vi "Count.vi"(0 "LV MDI in":refnum<class "LV MDI.lvclass">, 11 "error in (no error)":errorcluster) -> (4 "LV MDI out":refnum<class "LV MDI.lvclass">, 10 "Count":i32, 15 "error out":errorcluster)   [LabVIEW 2016, in "LV MDI.lvclass"]
doc: "Returns number of loaded vi."
uses:
  LV MDI.lvclass
  LV MDI.lvclass/LV MDI.ctl
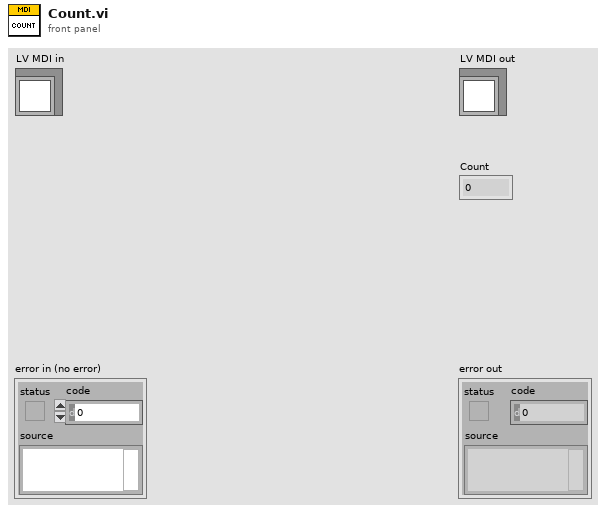
[diagram p1: front panel]
types:
  T1 = typedef "LV MDI.lvclass/Child Window Data.ctl" = cluster{"Child hWnd":u32, "UID":string, "vi reference":refnum<vi>, "Name":string}
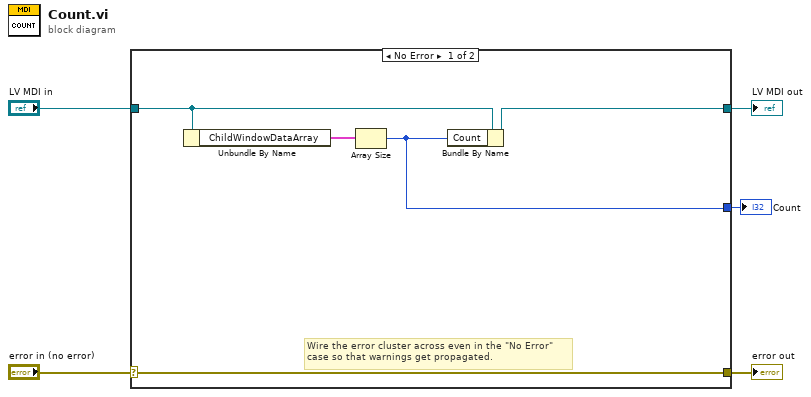
[diagram p0: block diagram]
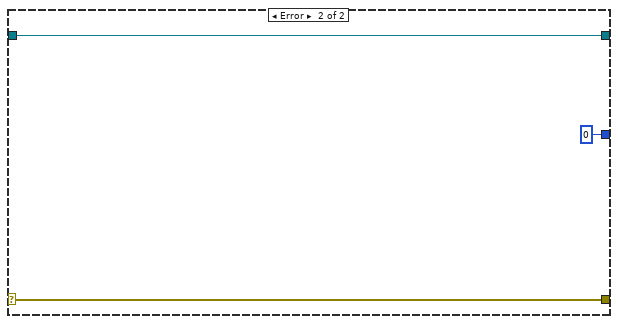
[diagram p2: hidden frame]
diagram:
  n1 = case shown="No Error" "error in (no error)" {
    selector: "error in (no error)" -> [w10 w13]
    tunnel: [w10 w13] -> w4
    tunnel: [w7 w12] -> w2
    tunnel: "LV MDI in" -> [w8 w12]
    tunnel: [w6 0] -> w1
    frame No Error {
      # "Wire the error cluster across even in the \"No Error\"\ncase so that warnings get propagated."
      n2 = Unbundle By Name(w8) -> ("ChildWindowDataArray"=w9:T1[])
      n3 = Array Size(array=w9) -> (size(s)=w6:i32)
      n4 = Bundle By Name(cluster=w8, "Count"=w6) -> (w7:refnum<class "LV MDI.lvclass">)
    }
    frame Error {
    }
  }
  "error out" <- w4
  "LV MDI out" <- w2
  "Count" <- w1
